vi "NumPromRequest.vi"() -> (0 "NumProm":u8=100)   [LabVIEW 2013]
panel:
  in  "Numeric":u8=99 max=99 step=1
  in  "OK Button":bool
  # "Introduce el nuevo número de promedios"
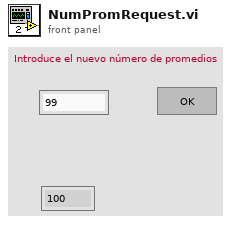
[diagram p1: front panel]
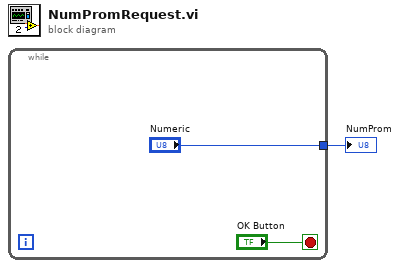
[diagram p0: block diagram]
diagram:
  n1 = while {
    tunnel: ["Numeric"] -> w1
    stop <- "OK Button" stop-if-true
  }
  "NumProm" <- w1
